vi "Execute.vi"(8 "error in (no error)":errorcluster, 10 "System In":refnum<class "abs_System.lvclass">, 11 "Node in":refnum<class "abs_Composite.lvclass">) -> (0 "error out":errorcluster, 1 "Status":T1, 2 "System Out":refnum<class "abs_System.lvclass">, 3 "Node out":refnum<class "abs_Composite.lvclass">)   [LabVIEW 2021, in "BT.lvlib" / "abs_Composite.lvclass"]
uses:
  abs_Composite.lvclass
  abs_Node/Status.ctl
  abs_System/abs_System.lvclass
  abs_Composite.lvclass/abs_Composite.ctl
  Properties/Read Index.vi
  abs_Node/abs_Node.lvclass
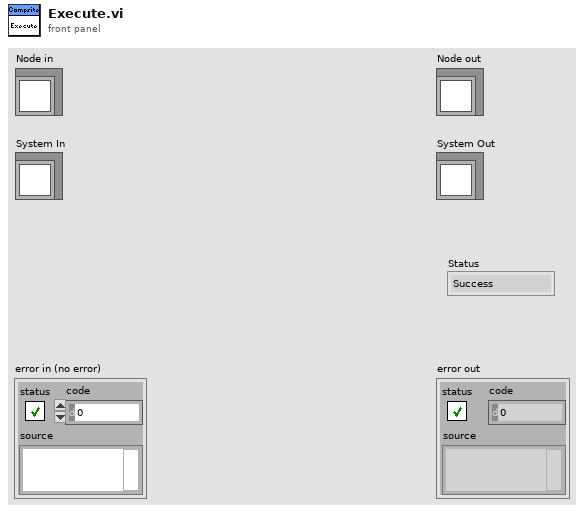
[diagram p1: front panel]
types:
  T1 = typedef "BT.lvlib/abs_Node.lvclass/Status.ctl" = enum16{"Success", "Failure", "Running"}
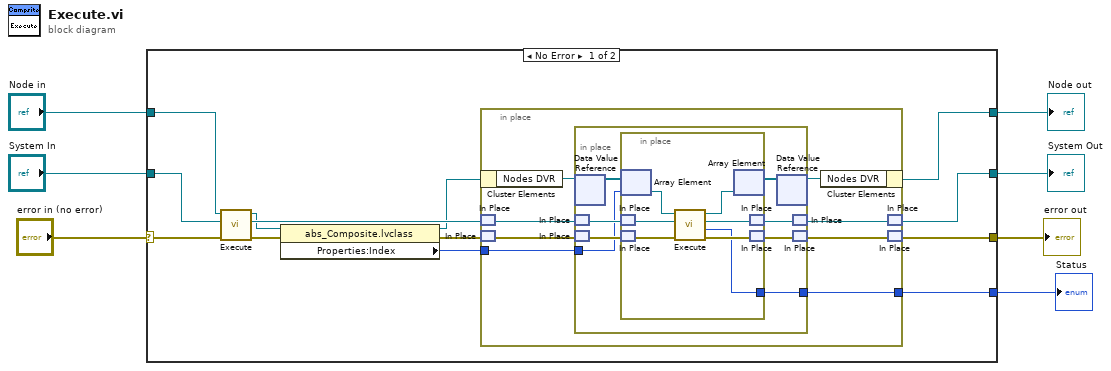
[diagram p0: block diagram]
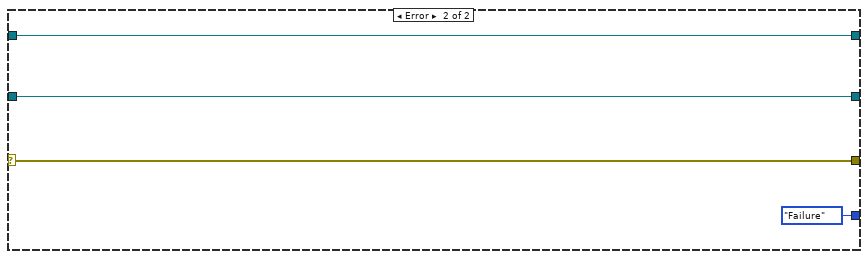
[diagram p2: hidden frame]
diagram:
  n1 = case shown="No Error" "error in (no error)" {
    selector: "error in (no error)" -> [w20 w45]
    tunnel: "System In" -> [w19 w46]
    tunnel: "Node in" -> [w18 w47]
    tunnel: [w17 w47] -> w4
    tunnel: [w15 w46] -> w3
    tunnel: [w14 w45] -> w2
    tunnel: [w13 Status."Failure" ("Status")] -> w1
    frame No Error {
      n2 = call-parent "Execute.vi"("error in (no error)"=w20, "System In"=w19, "Node in"=w18) -> ("error out"=w12:errorcluster, "System Out"=w16:refnum<class "abs_System.lvclass">, "Node out"=w10:refnum<class "abs_Composite.lvclass">)  [unwired: 5 in, 1 out]
      n3 = property class="abs_Composite.lvclass"(reference=w10, error in=w12) -> (reference out=w9:refnum<class "abs_Composite.lvclass">, error out=w11:errorcluster, "Properties:Index"=w8:i32)
      n4 = in-place {
        in-place-border: [w22] -> w13
        in-place-border: w8 -> [w21]
        n5 = in-place-cluster #1(w9) -> ("Nodes DVR"=w28:refnum<data-value>)
        n6 = in-place-match #2(w16) -> (w26:refnum<class "abs_System.lvclass">)
        n7 = in-place-match #3(w11) -> (w25:errorcluster)
        n8 = in-place {
          in-place-border: [w30] -> w22
          in-place-border: w21 -> [w29]
          n9 = in-place-dvr #4(w28) -> (w36:refnum<class "abs_Node.lvclass">[])  [unwired: 1 out]
          n10 = in-place-match #5(w26) -> (w34:refnum<class "abs_System.lvclass">)
          n11 = in-place-match #6(w25) -> (w33:errorcluster)
          n12 = in-place {
            in-place-border: [w37] -> w30
            n13 = in-place-array #7(w36, w29) -> (w43:refnum<class "abs_Node.lvclass">)
            n14 = in-place-match #8(w34) -> (w40:refnum<class "abs_System.lvclass">)
            n15 = in-place-match #9(w33) -> (w41:errorcluster)
            n16 = call-dynamic "Execute.vi"("error in (no error)"=w41, "System In"=w40, "Node in"=w43) -> ("error out"=w39:errorcluster, "Status"=w37:T1, "System Out"=w38:refnum<class "abs_System.lvclass">, "Node out"=w42:refnum<class "abs_Node.lvclass">)  [unwired: 5 in]
            n17 = in-place-array #7(w42) -> (w35:refnum<class "abs_Node.lvclass">[])  [unwired: 1 out]
            n18 = in-place-match #8(w38) -> (w32:refnum<class "abs_System.lvclass">)
            n19 = in-place-match #9(w39) -> (w31:errorcluster)
          }
          n20 = in-place-dvr #4(w35) -> (w27:refnum<data-value>)  [unwired: 1 out]
          n21 = in-place-match #5(w32) -> (w24:refnum<class "abs_System.lvclass">)
          n22 = in-place-match #6(w31) -> (w23:errorcluster)
        }
        n23 = in-place-cluster #1("Nodes DVR"=w27) -> (w17:refnum<class "abs_Composite.lvclass">)
        n24 = in-place-match #2(w24) -> (w15:refnum<class "abs_System.lvclass">)
        n25 = in-place-match #3(w23) -> (w14:errorcluster)
      }
    }
    frame Error {
    }
  }
  "error out" <- w2
  "Node out" <- w4
  "Status" <- w1
  "System Out" <- w3
